vi "Set Target Velocity.vi"(9 "Control Mode":T1 items=["PercentOutput"=0, "Position"=1, "Velocity"=2, "Current"=3, "Follower"=5, "MotionProfile"=6, "MotionMagic"=7, "MotionProfileArc"=10, "Disabled"=15], 10 "Input":cluster{"LF":dbl, "LB":dbl, "RF":dbl, "RB":dbl}, 11 "Swerve motors":cluster{"LF":T2, "LB":T2, "RF":T2, "RB":T2}) -> ()   [LabVIEW 2020]
uses:
  <vilib>/Rock Robotics/WPI/MotorControl/WPI_MotorControlDeviceRef.ctl
  <vilib>/Rock Robotics/WPI/MotorControl/WPI_MotorControlType.ctl
  <vilib>/Rock Robotics/SystemInterfaces/DIO/FPGA_DIOPWMChannel.ctl
  <vilib>/Rock Robotics/WPI/PWM/WPI_PWMDeadband.ctl
  <vilib>/Rock Robotics/SystemInterfaces/DIO/FPGA_DIOChannel.ctl
  <vilib>/Rock Robotics/WPI/ThirdParty/Phoenix-LabVIEW/Motor Controller/Controls/CTRE_Phoenix_MotorControl_ControlMode.ctl
  6b64e063-40b4-435e-b595-c1611d5f6bb1.vi
  <vilib>/Rock Robotics/WPI/ThirdParty/Phoenix-LabVIEW/Motor Controller/Get/CTRE_Phoenix_MotorController_GetSelectedSensorData.vi
panel:
  in  "Push PID":bool
  in  "Debug Mode":bool
  out "Drive \nErrors":cluster{dbl, dbl, dbl, dbl}(graph)
  in  "F":dbl
  in  "D":dbl
  in  "I":dbl
  in  "P":dbl
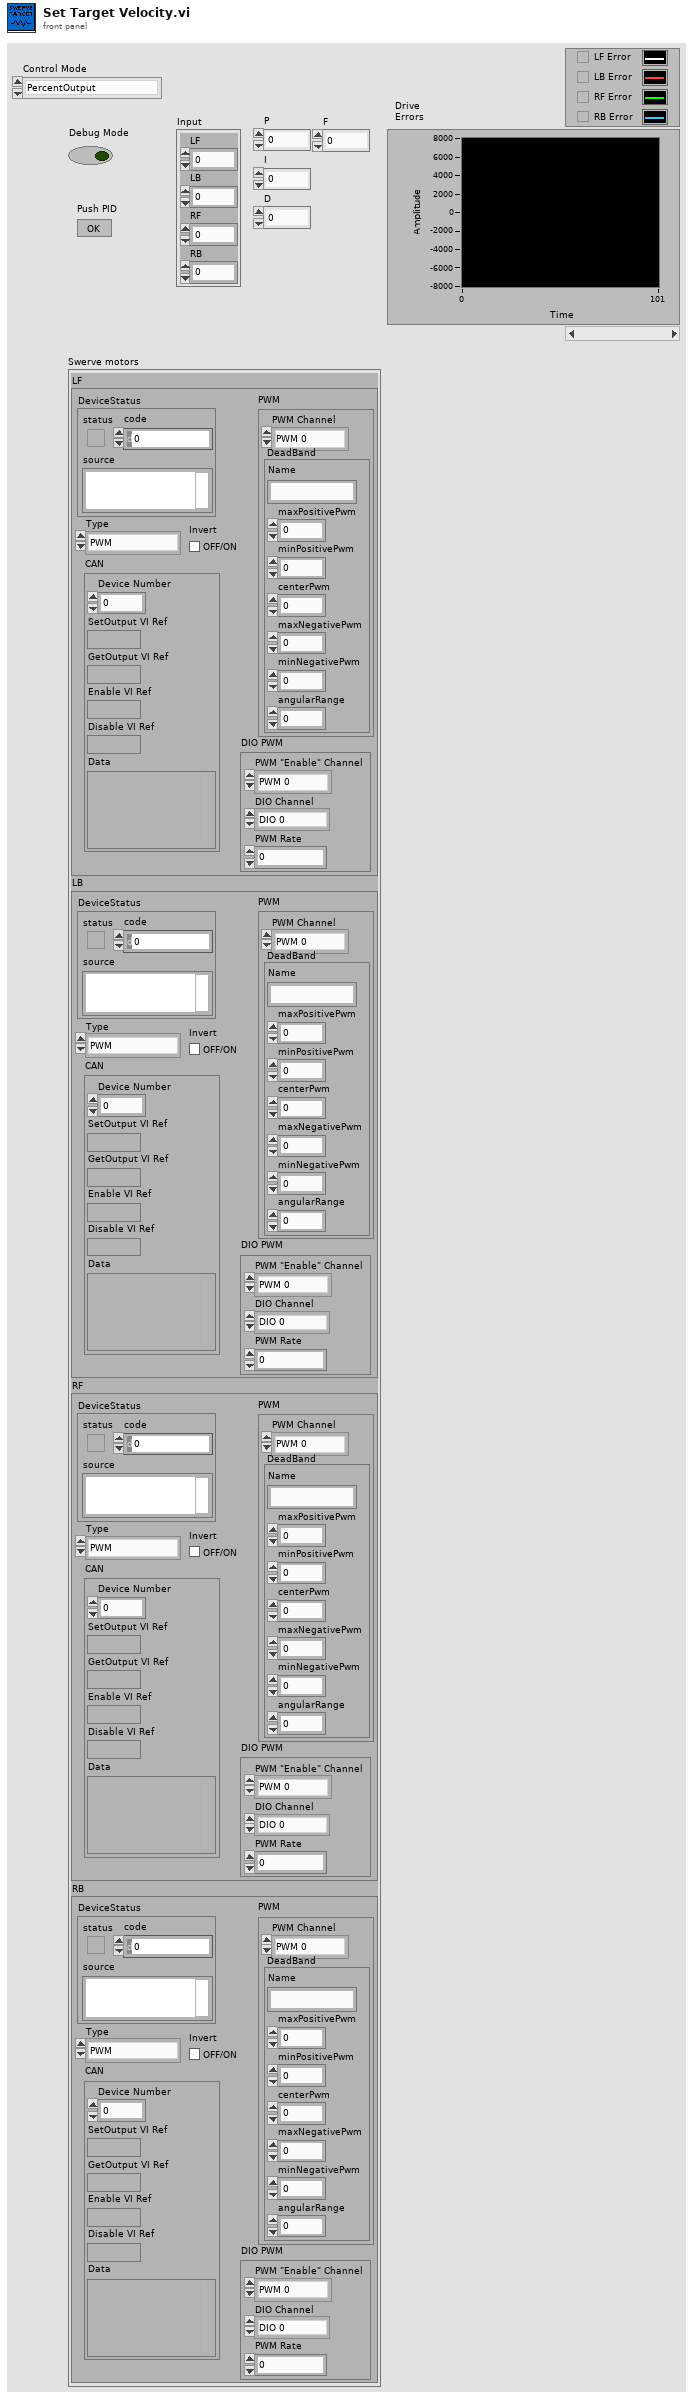
[diagram p1: front panel]
types:
  T1 = typedef "CTRE_Phoenix_MotorControl_ControlMode.ctl" = u16
  T2 = typedef "WPI_MotorControlDeviceRef.ctl" = cluster{"DeviceStatus":errorcluster, "Type":T3, "PWM":cluster{"PWM Channel":T4, "DeadBand":T5}, "CAN":cluster{"Device Number":u8, "SetOutput VI Ref":variant, "GetOutput VI Ref":variant, "Enable VI Ref":variant, "Disable VI Ref":variant, "Data":variant}, "Invert":bool, "DIO PWM":cluster{"PWM \"Enable\" Channel":T4, "DIOChannel":T6, "PWM Rate":dbl}}
  T3 = typedef "WPI_MotorControlType.ctl" = enum16{"PWM", "CAN", "DIO PWM"}
  T4 = typedef "FPGA_DIOPWMChannel.ctl" = enum8{"PWM 0", "PWM 1", "PWM 2", "PWM 3", "PWM 4", "PWM 5", "PWM 6", "PWM 7", "PWM 8", "PWM 9", "PWM MXP 0", "PWM MXP 1", "PWM MXP 2", "PWM MXP 3", "PWM MXP 4", "PWM MXP 5", "PWM MXP 6", "PWM MXP 7", "PWM MXP 8", "PWM MXP 9", "Invalid"}
  T5 = typedef "WPI_PWMDeadband.ctl" = cluster{"Name":string, "maxPositivePwm":i32, "minPositivePwm":i32, "centerPwm":i32, "maxNegativePwm":i32, "minNegativePwm":i32, "angularRange":u16}
  T6 = typedef "FPGA_DIOChannel.ctl" = enum8{"DIO 0", "DIO 1", "DIO 2", "DIO 3", "DIO 4", "DIO 5", "DIO 6", "DIO 7", "DIO 8", "DIO 9", "DIO MXP 0", "DIO MXP 1", "DIO MXP 2", "DIO MXP 3", "DIO MXP 4", "DIO MXP 5", "DIO MXP 6", "DIO MXP 7", "DIO MXP 8", "DIO MXP 9", "DIO MXP 10", "DIO MXP 11", "DIO MXP 12", "DIO MXP 13", "DIO MXP 14", "DIO MXP 15", "SPI Port CS1", "SPI Port CS2", "SPI Port CS3", "SPI Port MISO", "SPI Port MOSI", "Invalid"}
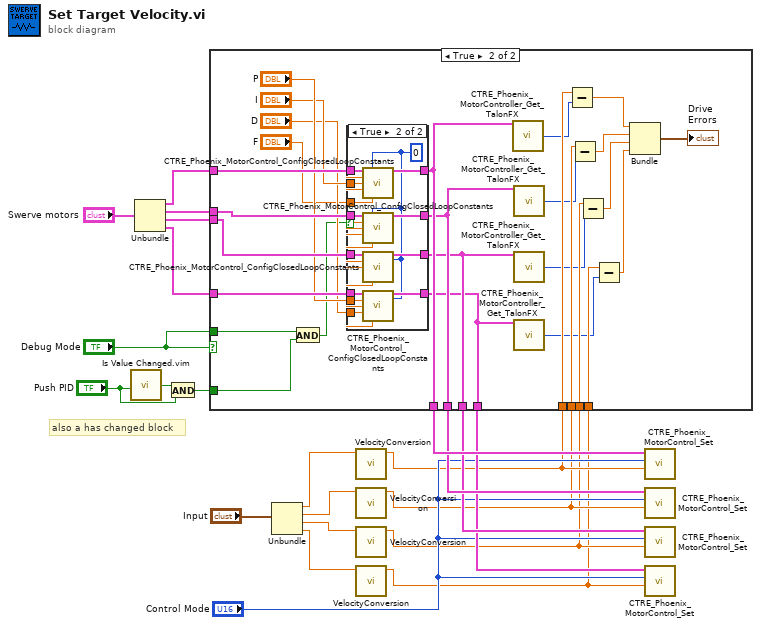
[diagram p0: block diagram]
diagram:
  # "also a has changed block"
  n1 = call "Is Value Changed.vim"("value"="Push PID") -> ("changed or first call?"=w2:bool)
  n2 = Unbundle("Swerve motors") -> ("LF"=w22:T2, "LB"=w21:T2, "RF"=w20:T2, "RB"=w19:T2)
  n3 = And(x=w2, y="Push PID") -> (x .and. y?=w3:bool)
  n4 = Unbundle("Input") -> ("LF"=w17:dbl, "LB"=w16:dbl, "RF"=w15:dbl, "RB"=w14:dbl)
  n5 = call "VelocityConversion.vi"("Velocity (ft/s)"=w17) -> ("Velocity (ticks/ds)"=w8:dbl)  [unwired: 10 in]
  n6 = call "VelocityConversion.vi"("Velocity (ft/s)"=w16) -> ("Velocity (ticks/ds)"=w7:dbl)  [unwired: 10 in]
  n7 = call "VelocityConversion.vi"("Velocity (ft/s)"=w15) -> ("Velocity (ticks/ds)"=w6:dbl)  [unwired: 10 in]
  n8 = call "VelocityConversion.vi"("Velocity (ft/s)"=w14) -> ("Velocity (ticks/ds)"=w5:dbl)  [unwired: 10 in]
  n9 = case shown="True" "Debug Mode" {
    tunnel: w22 -> [w27 w55]
    tunnel: w21 -> [w26 w54]
    tunnel: w20 -> [w25 w53]
    tunnel: w19 -> [w24 w52]
    tunnel: [w27 w47] -> w13
    tunnel: [w26 w46] -> w12
    tunnel: [w25 w45] -> w11
    tunnel: [w24 w44] -> w10
    tunnel: w8 -> [_ w43]
    tunnel: w7 -> [_ w40]
    tunnel: w6 -> [_ w37]
    tunnel: w5 -> [_ w34]
    tunnel: "Debug Mode" -> [_ w29]
    tunnel: w3 -> [_ w28]
    frame False {
    }
    frame True {
      n10 = And(x=w29, y=w28) -> (x .and. y?=w30:bool)
      n11 = case shown="True" w30 {
        tunnel: w55 -> [w59 w72]
        tunnel: w54 -> [w58 w71]
        tunnel: w53 -> [w57 w70]
        tunnel: w52 -> [w56 w69]
        tunnel: "P" -> [_ w68]
        tunnel: "I" -> [_ w67]
        tunnel: "D" -> [_ w66]
        tunnel: "F" -> [_ w65]
        tunnel: [w59 w64] -> w47
        tunnel: [w58 w63] -> w46
        tunnel: [w57 w62] -> w45
        tunnel: [w56 w61] -> w44
        frame False {
        }
        frame True {
          w60 = 0 ("slotIdx")
          n12 = call <vilib>:"CTRE_Phoenix_MotorControl_ConfigClosedLoopConstants.vi"("PhoenixMotorControlDevRef"=w72, "slotIdx"=w60, "P"=w68, "I"=w67, "D"=w66, "F"=w65) -> ("PhoenixMotorControlDevRef"=w64:T2)  [unwired: 8 in, 1 out]
          n13 = call <vilib>:"CTRE_Phoenix_MotorControl_ConfigClosedLoopConstants.vi"("PhoenixMotorControlDevRef"=w71, "slotIdx"=w60, "P"=w68, "I"=w67, "D"=w66, "F"=w65) -> ("PhoenixMotorControlDevRef"=w63:T2)  [unwired: 8 in, 1 out]
          n14 = call <vilib>:"CTRE_Phoenix_MotorControl_ConfigClosedLoopConstants.vi"("PhoenixMotorControlDevRef"=w70, "slotIdx"=w60, "P"=w68, "I"=w67, "F"=w65) -> ("PhoenixMotorControlDevRef"=w62:T2)  [unwired: 9 in, 1 out]
          n15 = call <vilib>:"CTRE_Phoenix_MotorControl_ConfigClosedLoopConstants.vi"("PhoenixMotorControlDevRef"=w69, "slotIdx"=w60, "P"=w68, "I"=w67, "D"=w66, "F"=w65) -> ("PhoenixMotorControlDevRef"=w61:T2)  [unwired: 8 in, 1 out]
        }
      }
      n16 = call-poly <vilib>:"CTRE_Phoenix_MotorController_Get_TalonFX.vi"("PhoenixMotorControlDevRef"=w47) -> ("Velocity (Raw Sensor Units per 100 ms)"=w42:i32)  [unwired: 11 in, 3 out]
      n17 = call-poly <vilib>:"CTRE_Phoenix_MotorController_Get_TalonFX.vi"("PhoenixMotorControlDevRef"=w46) -> ("Velocity (Raw Sensor Units per 100 ms)"=w39:i32)  [unwired: 11 in, 3 out]
      n18 = call-poly <vilib>:"CTRE_Phoenix_MotorController_Get_TalonFX.vi"("PhoenixMotorControlDevRef"=w45) -> ("Velocity (Raw Sensor Units per 100 ms)"=w36:i32)  [unwired: 11 in, 3 out]
      n19 = call-poly <vilib>:"CTRE_Phoenix_MotorController_Get_TalonFX.vi"("PhoenixMotorControlDevRef"=w44) -> ("Velocity (Raw Sensor Units per 100 ms)"=w33:i32)  [unwired: 11 in, 3 out]
      n20 = Subtract(x=w43, y=w42) -> (x-y=w41:dbl)
      n21 = Subtract(x=w40, y=w39) -> (x-y=w38:dbl)
      n22 = Subtract(x=w37, y=w36) -> (x-y=w35:dbl)
      n23 = Subtract(x=w34, y=w33) -> (x-y=w32:dbl)
      n24 = Bundle(w41, w38, w35, w32) -> (→"Drive \nErrors":cluster{dbl, dbl, dbl, dbl})  [unwired: 1 in]
    }
  }
  n25 = call <vilib>:"CTRE_Phoenix_MotorControl_Set.vi"("Output"=w8, "Control Mode"="Control Mode", "PhoenixMotorControlDevRef"=w13) -> ()  [unwired: 7 in, 2 out]
  n26 = call <vilib>:"CTRE_Phoenix_MotorControl_Set.vi"("Output"=w7, "Control Mode"="Control Mode", "PhoenixMotorControlDevRef"=w12) -> ()  [unwired: 7 in, 2 out]
  n27 = call <vilib>:"CTRE_Phoenix_MotorControl_Set.vi"("Output"=w6, "Control Mode"="Control Mode", "PhoenixMotorControlDevRef"=w11) -> ()  [unwired: 7 in, 2 out]
  n28 = call <vilib>:"CTRE_Phoenix_MotorControl_Set.vi"("Output"=w5, "Control Mode"="Control Mode", "PhoenixMotorControlDevRef"=w10) -> ()  [unwired: 7 in, 2 out]
